vi "USBTC08OpenUnit.vi"(8 "error in (no error)":errorcluster) -> (0 "error out":errorcluster, 3 "Handle out":i16)   [LabVIEW 2009]
uses:
  usbtc08.dll
panel:
  out "Handle":i16
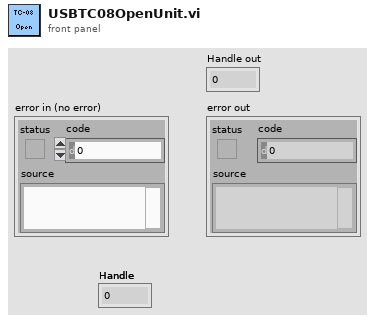
[diagram p1: front panel]
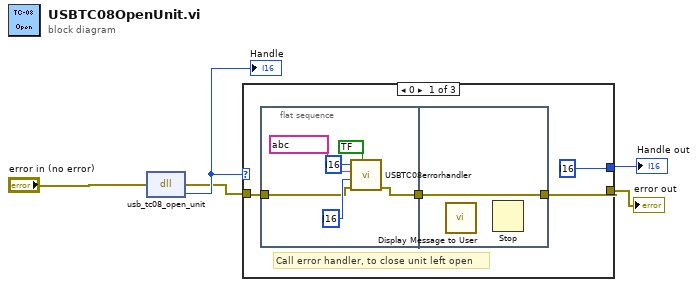
[diagram p0: block diagram]
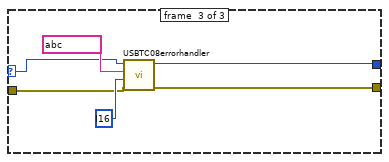
[diagram p3: hidden frame]
diagram:
  n1 = dll-call lib="usbtc08.dll" fn="usb_tc08_open_unit" label="OpenUnit"(error in="error in (no error)") -> (error out=w3:errorcluster, "Handle"=w5:i16)  [unwired: 2 in, 1 out]
  "Handle" <- w5
  n2 = case shown="0" w5 {
    selector: w5 -> [_ w18 w20]
    tunnel: [i16 ? ("Handle") w18 w19] -> w4
    tunnel: w3 -> [w8 w17 w22]
    tunnel: [w7 w17 w21] -> w1
    frame #0 {
      # "Call error handler, to close unit left open"
      n3 = flat-sequence {
        tunnel: w8 -> [w13]
        tunnel: [w12] -> w6
        tunnel: [w16] -> w7
        tunnel: w6 -> [w16]
        frame #0 {
          n4 = call "USBTC08errorhandler.vi"("Close unit"=bool ?, "error in (no error)"=w13, "Return"=i16 ?, "API function"=string ?, "Handle in"=i16 ?) -> ("error out"=w12:errorcluster)  [unwired: 5 in, 1 out]
        }
        frame #1 {
          n5 = call "Display Message to User"() -> ()  [unwired: 10 in, 2 out]
          n6 = Stop() -> ()  [unwired: 1 in]
        }
      }
    }
    frame #1 {
      # "Any valid handle value >0"
    }
    frame #2 {
      n7 = call "USBTC08errorhandler.vi"("error in (no error)"=w22, "Return"=i16 ?, "API function"=string ?, "Handle in"=w20) -> ("error out"=w21:errorcluster, "Handle out"=w19:i16)  [unwired: 6 in]
    }
  }
  "Handle out" <- w4
  "error out" <- w1
